vi "Send Views User Event.vi"(8 "error in (no error)":errorcluster, 11 "GUI Container in":refnum<class "GUI Container.lvclass">) -> (0 "error out":errorcluster, 3 "GUI Container out":refnum<class "GUI Container.lvclass">)   [LabVIEW 2023, in "GUI Views.lvlib" / "GUI Container.lvclass"]
uses:
  GUI Container.lvclass
  GUI Container.lvclass/GUI Container.ctl
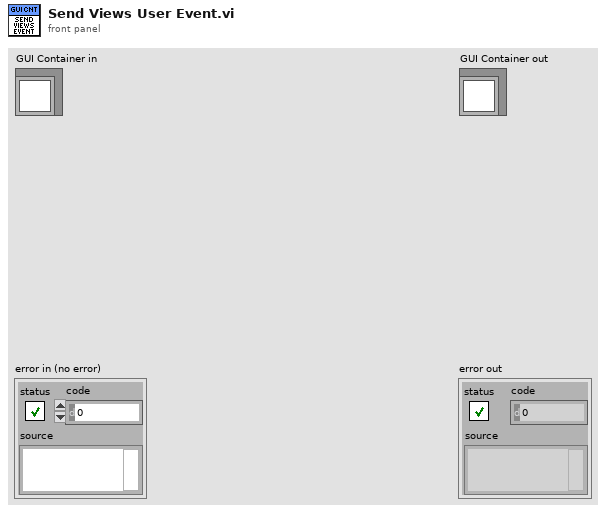
[diagram p1: front panel]
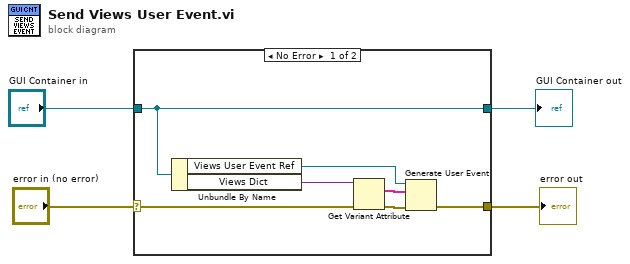
[diagram p0: block diagram]
diagram:
  n1 = case shown="No Error" "error in (no error)" {
    selector: "error in (no error)" -> [w9 w13]
    tunnel: [w5 w13] -> w3
    tunnel: [w11 w12] -> w1
    tunnel: "GUI Container in" -> [w11 w12]
    frame No Error {
      n2 = Unbundle By Name(w11) -> ("Views User Event Ref"=w6:refnum<user-event>, "Views Dict"=w10:variant)
      n3 = Get Variant Attribute(Variant=w10, error in=w9) -> (names=w8:string[], error out=w7:errorcluster)  [unwired: 2 in, 2 out]
      n4 = Generate User Event(user event=w6, event data cluster=w8, error in=w7) -> (error out=w5:errorcluster)  [unwired: 1 in, 1 out]
    }
    frame Error {
    }
  }
  "error out" <- w3
  "GUI Container out" <- w1
